vi "Step.vi"(8 "error in (no error)":errorcluster, 9 "LTS Current (A)":dbl, 10 "HTS Current (A)":dbl, 11 "CurrentToField in":refnum<class "CurrentToField.lvclass">) -> (0 "error out":errorcluster, 2 "Field (T)":dbl, 3 "CurrentToField out":refnum<class "CurrentToField.lvclass">)   [LabVIEW 2019, in "CurrentToField.lvclass"]
uses:
  CurrentToField.lvclass
  CurrentToField.lvclass/CurrentToField.ctl
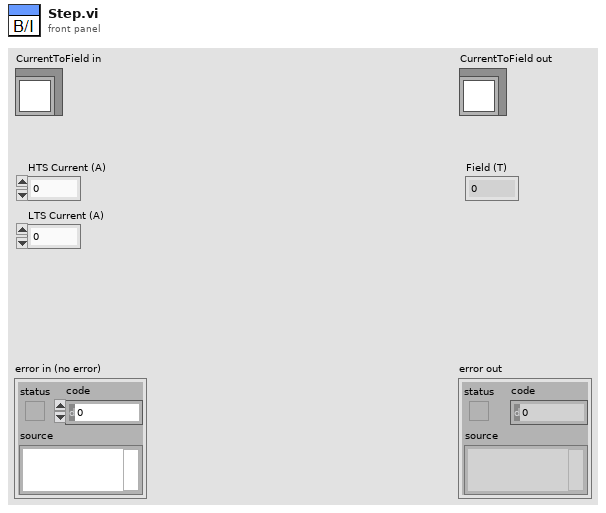
[diagram p1: front panel]
types:
  T1 = cluster{"HTS B_I0":dbl, "LTS B_I0":dbl, "HTS Bmax":dbl, "LTS Bmax":dbl, "Max combined rate (T/min)":dbl}
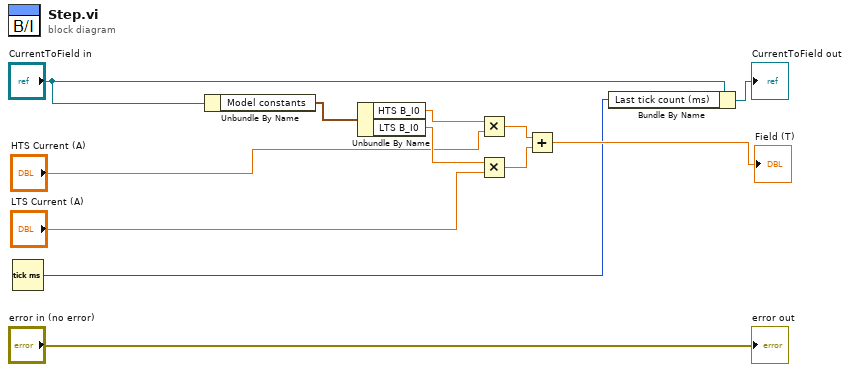
[diagram p0: block diagram]
diagram:
  n1 = Tick Count (ms)() -> (millisecond timer value=w1:u32)
  n2 = Unbundle By Name("CurrentToField in") -> ("Model constants"=w10:T1)
  n3 = Unbundle By Name(w10) -> ("HTS B_I0"=w9:dbl, "LTS B_I0"=w8:dbl)
  n4 = Multiply(x=w9, y="HTS Current (A)") -> (x*y=w7:dbl)
  n5 = Multiply(x=w8, y="LTS Current (A)") -> (x*y=w6:dbl)
  n6 = Add(x=w7, y=w6) -> (x+y=→"Field (T)":dbl)
  n7 = Bundle By Name(cluster="CurrentToField in", "Last tick count (ms)"=w1) -> (→"CurrentToField out":refnum<class "CurrentToField.lvclass">)
  "error out" <- "error in (no error)"
